vi "Read TCP Message.vi"(8 "error in (no error)":errorcluster, 11 "TCP Network Connection in":refnum<k5>) -> (0 "error out":errorcluster, 2 "data out":string, 3 "connection ID out":refnum<k5>)   [LabVIEW 2019]
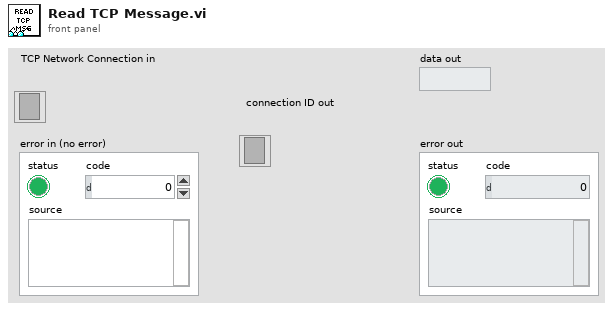
[diagram p1: front panel]
types:
  T1 = enum16{"Standard", "Buffered", "CRLF", "Immediate"}
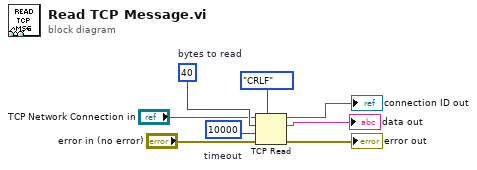
[diagram p0: block diagram]
diagram:
  w3 = 10000  # timeout
  w5 = 40  # bytes to read
  n1 = TCP Read(connection ID="TCP Network Connection in", bytes to read=w5, error in (no error)="error in (no error)", 7:T1."CRLF" ("mode (standard)"), 9:w3) -> (connection ID out=→"connection ID out":refnum<k5>, data out=→"data out":string, error out=→"error out":errorcluster)
